vi "master slave race around.vi"() -> ()   [LabVIEW 2012]
panel:
  in  "Master 2":bool
  in  "Master 1":bool
  out "latest notification 2":dbl
  out "latest notification":dbl
  in  "Master 2":dbl
  in  "Master 1":dbl
  # "Stop used to send notification from respective master"
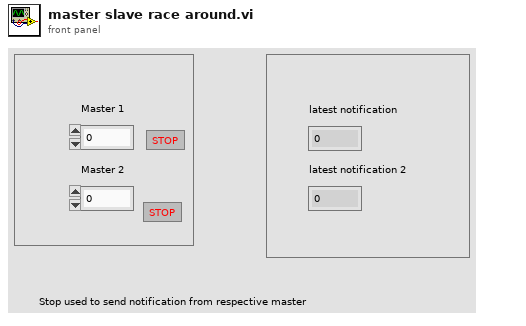
[diagram p1: front panel]
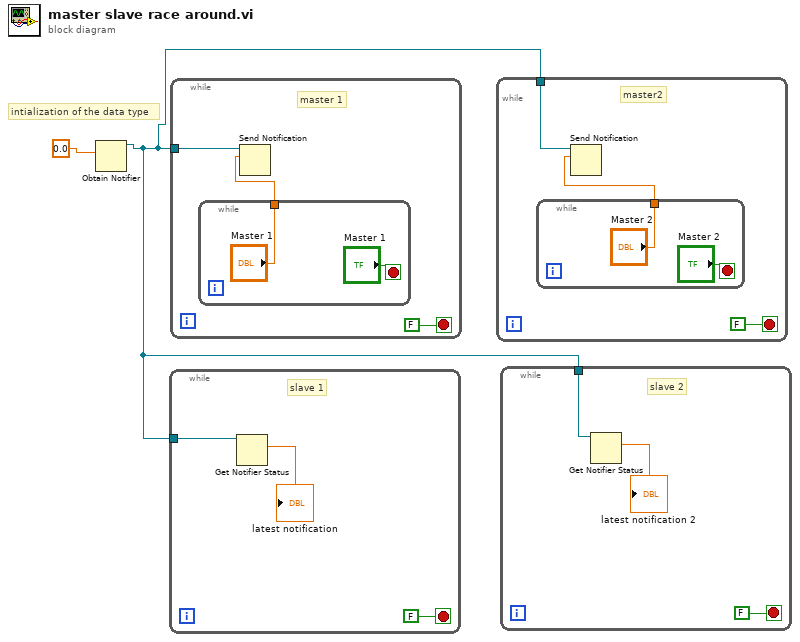
[diagram p0: block diagram]
diagram:
  # "intialization of the data type"
  n1 = Obtain Notifier(notification data type=0.0 ("Numeric 2")) -> (notifier out=w1:refnum<notifier>)  [unwired: 3 in, 2 out]
  n2 = while {
    tunnel: w1 -> [w4]
    stop <- FALSE stop-if-true
    # "slave 1"
    n3 = Get Notifier Status(notifier=w4) -> (current notification=→"latest notification":dbl)  [unwired: 1 in, 4 out]
  }
  n4 = while {
    tunnel: w1 -> [w7]
    stop <- FALSE stop-if-true
    # "master 1"
    n5 = while {
      tunnel: ["Master 1"] -> w6
      stop <- "Master 1" stop-if-true
    }
    n6 = Send Notification(notification=w6, notifier=w7) -> ()  [unwired: 1 in, 2 out]
  }
  n7 = while {
    tunnel: w1 -> [w12]
    stop <- FALSE stop-if-true
    # "master2"
    n8 = while {
      tunnel: ["Master 2"] -> w11
      stop <- "Master 2" stop-if-true
    }
    n9 = Send Notification(notification=w11, notifier=w12) -> ()  [unwired: 1 in, 2 out]
  }
  n10 = while {
    tunnel: w1 -> [w17]
    stop <- FALSE stop-if-true
    # "slave 2"
    n11 = Get Notifier Status(notifier=w17) -> (current notification=→"latest notification 2":dbl)  [unwired: 1 in, 4 out]
  }
